vi "16路数字量输入.vi"(9 "第几组数据":i32, 11 "CAN端口":u16) -> (2 "成功?":bool)   [LabVIEW 2010]
panel:
  # "从1开始"
  # "从1开始"
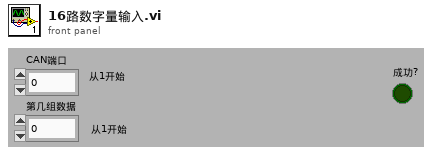
[diagram p1: front panel]
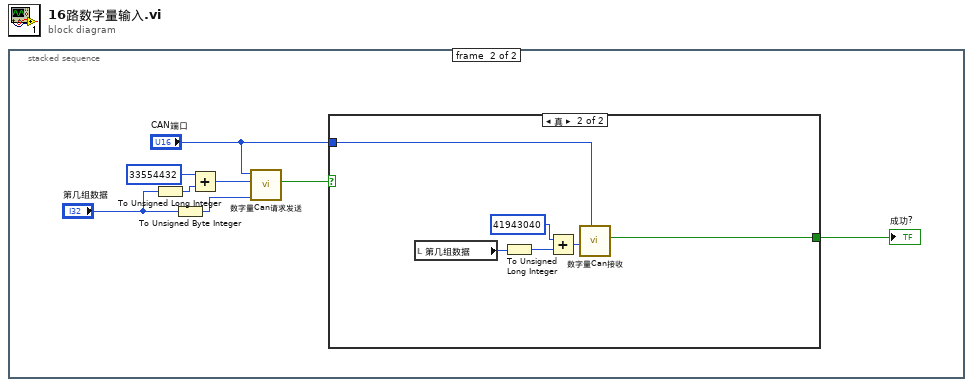
[diagram p0: block diagram]
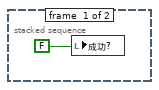
[diagram p2: hidden frame]
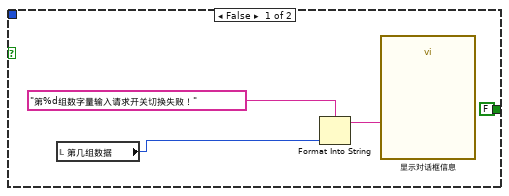
[diagram p3: hidden frame]
diagram:
  n1 = stacked-sequence {
    frame #0 {
      n2 = local write "成功?"(FALSE) -> ()
    }
    frame #1 {
      n3 = To Unsigned Long Integer(number="第几组数据") -> (unsigned 32bit integer=w6:u32)
      n4 = To Unsigned Byte Integer(number="第几组数据") -> (unsigned 8bit integer=w3:u8)
      n5 = Add(x=u32 33554432 ("CANPort"), y=w6) -> (x+y=w5:u32)
      n6 = call "数字量Can请求发送.vi"("第几组数据"=w3, "CANID"=w5, "CANPort"="CAN端口") -> ("发送成功?"=w2:bool)  [unwired: 8 in]
      n7 = case shown="真" w2 {
        tunnel: "CAN端口" -> [_ w19]
        tunnel: [FALSE w14] -> w9
        frame False {
          n8 = local read "第几组数据"() -> (w13:i32)
          n9 = Format Into String(format string="第%d组数字量输入请求开关切换失败！", w13) -> (resulting string=w12:string)  [unwired: 2 in, 1 out]
          n10 = call "显示对话框信息"("Message"=w12) -> ()  [unwired: 9 in, 2 out]
        }
        frame True {
          n11 = local read "第几组数据"() -> (w16:i32)
          n12 = To Unsigned Long Integer(number=w16) -> (unsigned 32bit integer=w15:u32)
          n13 = Add(x=u32 41943040 ("CANPort"), y=w15) -> (x+y=w17:u32)
          n14 = call "数字量Can接收.vi"("CANPort"=w19, "匹配CANID"=w17) -> ("成功？"=w14:bool)  [unwired: 8 in, 1 out]
        }
      }
      "成功?" <- w9
    }
  }
